vi "Write Ref No_.vi"(8 "error in (no error)":errorcluster, 10 "Ref No.":u32, 11 "AlessiRel6100 in":refnum<class "AlessiRel6100.lvclass">) -> (0 "error out":errorcluster, 3 "AlessiRel6100 out":refnum<class "AlessiRel6100.lvclass">)   [LabVIEW 2013, in "AlessiRel6100.lvclass"]
uses:
  AlessiRel6100.lvclass
  AlessiRel6100.lvclass/AlessiRel6100.ctl
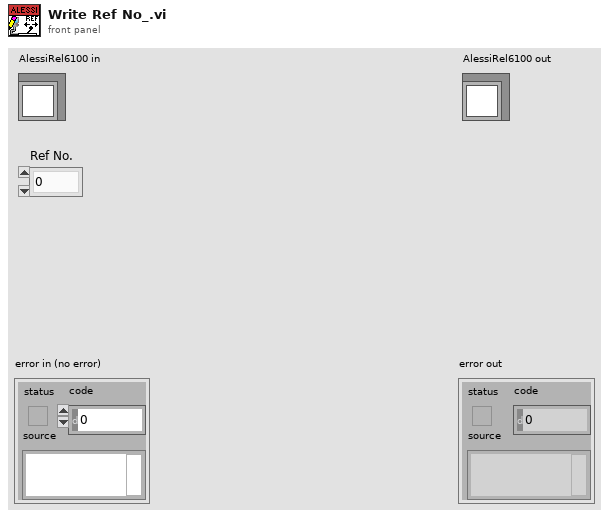
[diagram p1: front panel]
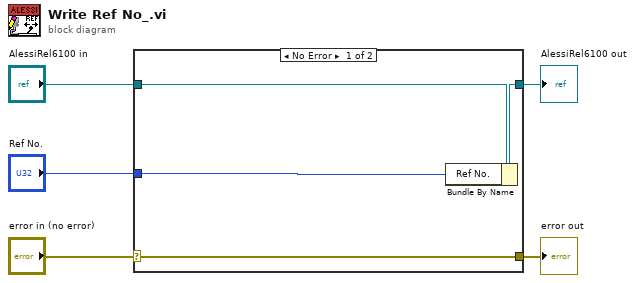
[diagram p0: block diagram]
diagram:
  n1 = case shown="No Error" "error in (no error)" {
    selector: "error in (no error)" -> [w9 w10]
    tunnel: [w9 w10] -> w4
    tunnel: [w7 w11] -> w2
    tunnel: "AlessiRel6100 in" -> [w8 w11]
    tunnel: "Ref No." -> [w6 _]
    frame No Error {
      n2 = Bundle By Name(cluster=w8, "Ref No."=w6) -> (w7:refnum<class "AlessiRel6100.lvclass">)
    }
    frame Error {
    }
  }
  "error out" <- w4
  "AlessiRel6100 out" <- w2
